vi "Betonauswahl.vi"(8 "error in (no error)":errorcluster) -> (0 "error out":errorcluster)   [LabVIEW 2023]
doc: "Dieses Vi ließt das config file für die Betonsorten und errechnet den Preis pro Menge\nerstellt: Tim Pusterhofer\nDatum 12.11.2025"
uses:
  CONTROLS/Betonauswahl.ctl
  <vilib>/Utility/miscctls.llb/LVRectTypeDef.ctl
panel:
  out "Preis":dbl
  in  "Enum":T1
  in  "Menge":dbl
  in  "Reserve Schalter 3":bool
  in  "Reserve Schalter 2":bool
  in  "Reserve Schalter":bool
  in  "Daten speichern":bool
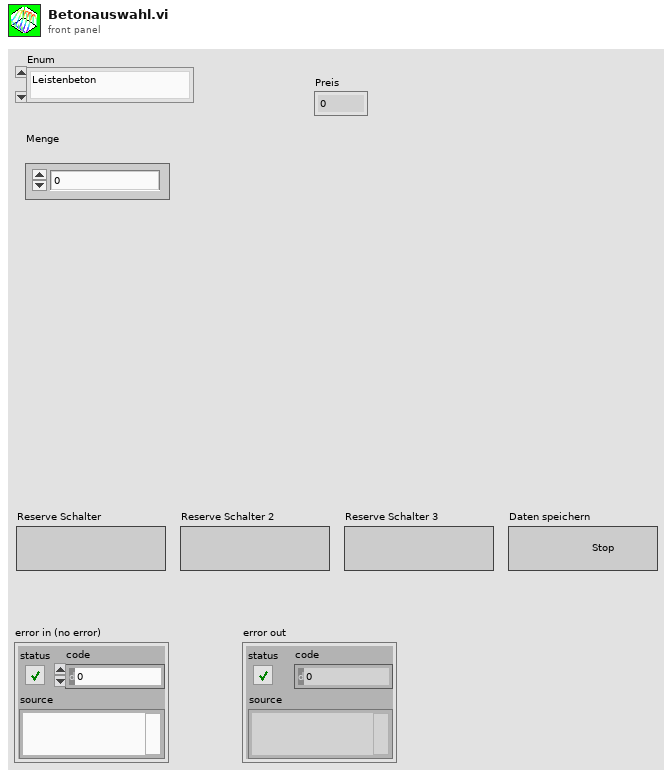
[diagram p1: front panel]
types:
  T1 = typedef "Betonauswahl.ctl" = enum16{"Leistenbeton", "Erdfeuchter Beton", "Beton", "ERdfeuchter Starker Beton", "Starker Beton", "Bet"}
  T2 = typedef "LVRectTypeDef.ctl" = cluster{"Left":i16, "Top":i16, "Right":i16, "Bottom":i16}
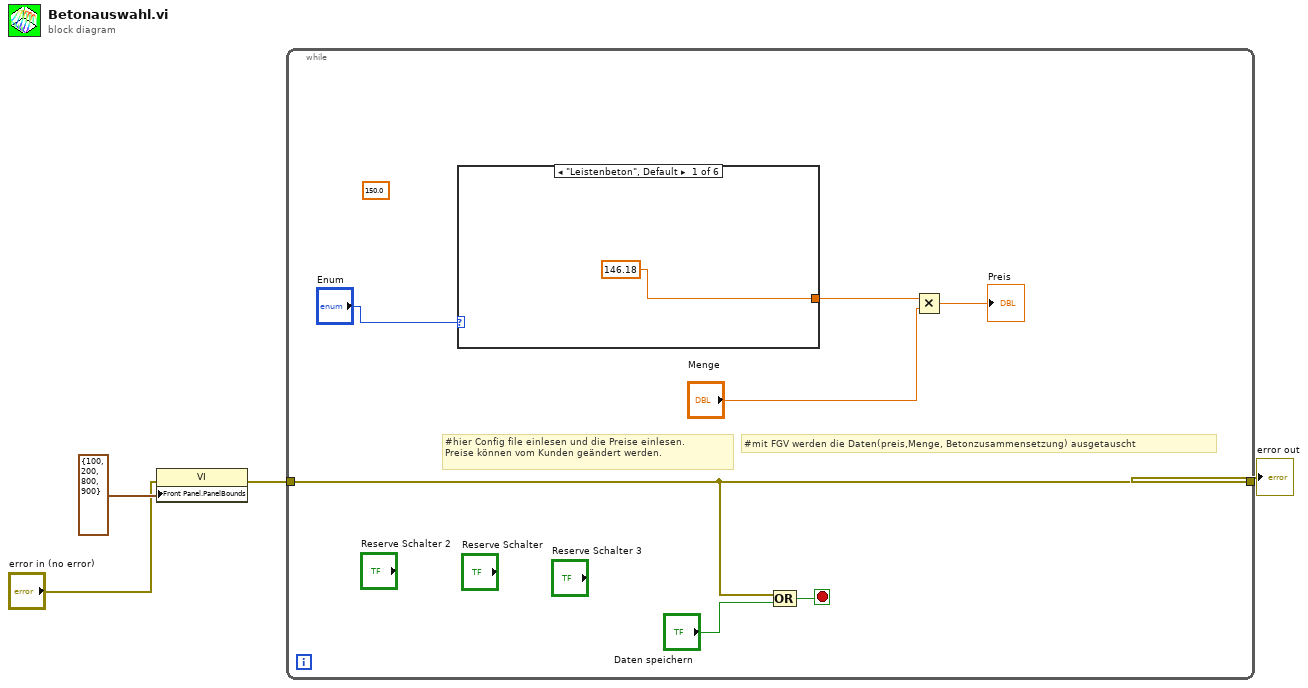
[diagram p0: block diagram]
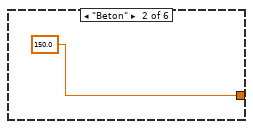
[diagram p2: hidden frame]
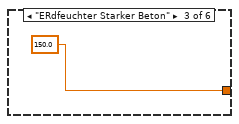
[diagram p3: hidden frame]
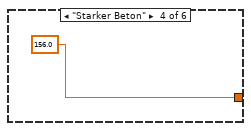
[diagram p4: hidden frame]
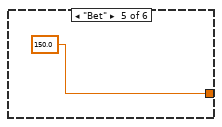
[diagram p5: hidden frame]
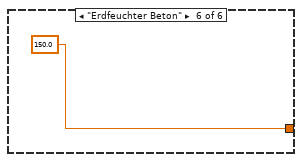
[diagram p6: hidden frame]
diagram:
  n1 = property class="VI"(error in="error in (no error)", "Front Panel.PanelBounds"=T2 {"Left"=100, "Top"=200, "Right"=800, "Bottom"=900} ("Front Panel Window:Panel Bounds")) -> (error out=w1:errorcluster)  [unwired: 1 in, 1 out]
  n2 = while {
    tunnel: [w10] -> w4
    tunnel: w1 -> [w10]
    stop <- w9 stop-if-true
    (unwired) 150.0
    # "#mit FGV werden die Daten(preis,Menge, Betonzusammensetzung) ausgetauscht"
    # "#hier Config file einlesen und die Preise einlesen.\nPreise können vom Kunden geändert werden."
    n3 = case shown="\"Leistenbeton\", Default" "Enum" {
      tunnel: [146.18 150.0 150.0 156.0 150.0 150.0] -> w6
      frame "Leistenbeton", Default {
      }
      frame "Beton" {
      }
      frame "ERdfeuchter Starker Beton" {
      }
      frame "Starker Beton" {
      }
      frame "Bet" {
      }
      frame "Erdfeuchter Beton" {
      }
    }
    n4 = Compound Arithmetic op=OR(w10, "Daten speichern") -> (w9:bool)
    n5 = Multiply(x=w6, y="Menge") -> (x*y=→"Preis":dbl)
  }
  "error out" <- w4
